vi "Set JSON Data.vi"(8 "error in (no error)":errorcluster, 10 "JSON Data":string, 11 "LVUnit Test Case in":refnum<class "LVUnit Test Case.lvclass">) -> (0 "error out":errorcluster, 3 "LVUnit Test Case out":refnum<class "LVUnit Test Case.lvclass">)   [LabVIEW 2017, in "LVUnit Test Case.lvclass"]
uses:
  LVUnit Test Case.lvclass
  LVUnit Test Case.lvclass/LVUnit Test Case.ctl
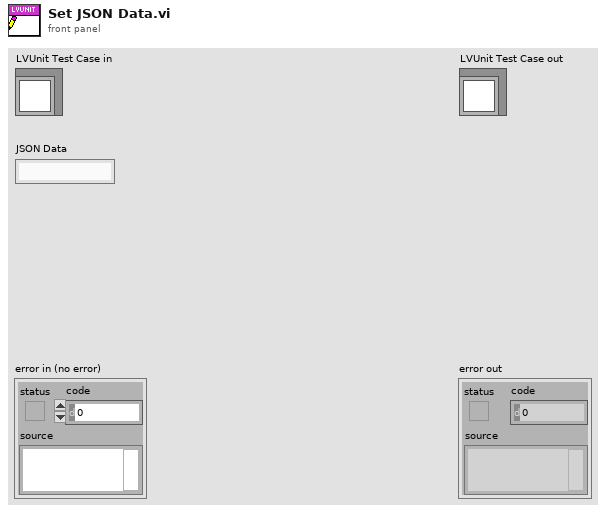
[diagram p1: front panel]
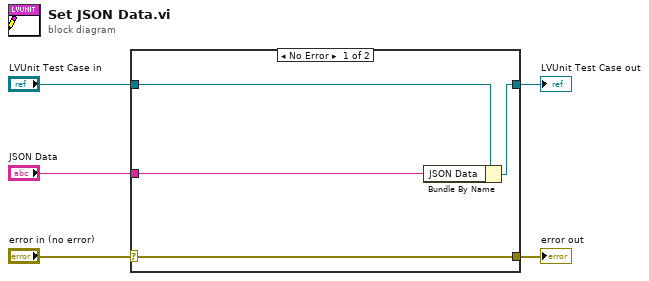
[diagram p0: block diagram]
diagram:
  n1 = case shown="No Error" "error in (no error)" {
    selector: "error in (no error)" -> [w9 w10]
    tunnel: [w9 w10] -> w4
    tunnel: [w7 w11] -> w2
    tunnel: "LVUnit Test Case in" -> [w8 w11]
    tunnel: "JSON Data" -> [w6 _]
    frame No Error {
      n2 = Bundle By Name(cluster=w8, "JSON Data"=w6) -> (w7:refnum<class "LVUnit Test Case.lvclass">)
    }
    frame Error {
    }
  }
  "error out" <- w4
  "LVUnit Test Case out" <- w2
